vi "Access Privilege_String Encrypt Decrypt.vi"(9 "Encrypted In":u8[][][](array[numeric]), 10 "2D String Data":string[][](array[string])=[["Administrator", "Admin", "Administrator"], ["1", "1", "Administrator"], ["2", "2", "User"]], 11 "Action":enum16{"Encrypt", "Decrypt"}(ring)) -> (1 "Decrypted Out":string[][](array[string]), 2 "Encrypted Out":u8[][][](array[numeric]))   [LabVIEW 2023, in "GUI.lvlib"]
uses:
  GUI.lvlib
  <vilib>/Utility/error.llb/Trim Whitespace One-Sided.vi
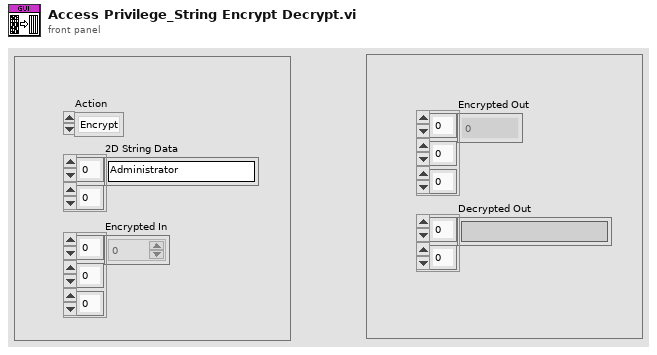
[diagram p1: front panel]
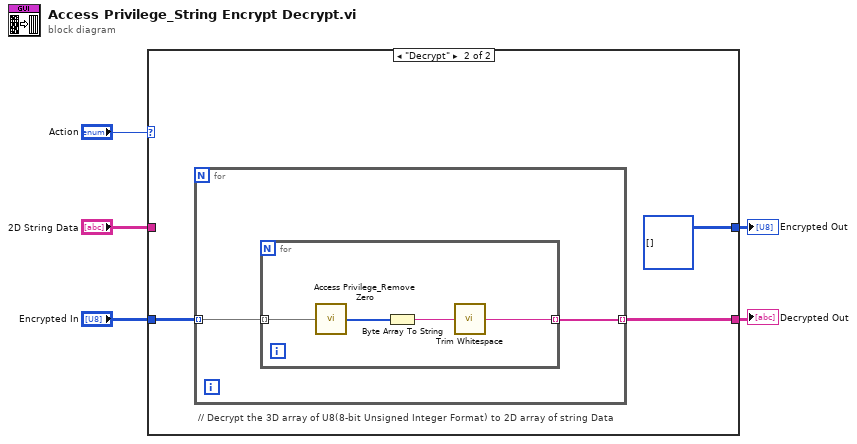
[diagram p0: block diagram]
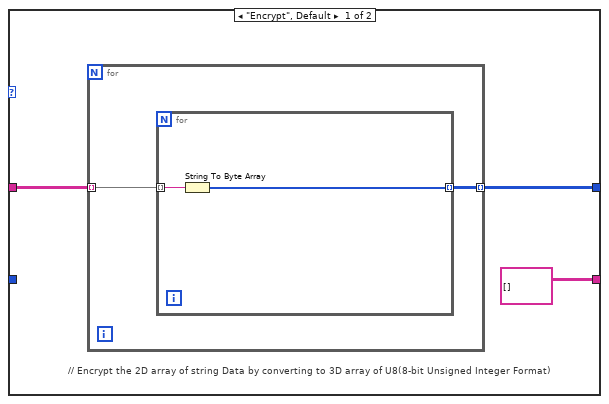
[diagram p2: hidden frame]
diagram:
  n1 = case shown="\"Decrypt\"" "Action" {
    tunnel: "2D String Data" -> [w8 _]
    tunnel: [w7 u8[][][] [] ("unsigned byte array")] -> w3
    tunnel: "Encrypted In" -> [_ w14]
    tunnel: [string[][] [] w13] -> w1
    frame "Encrypt", Default {
      # "// Encrypt the 2D array of string Data by converting to 3D array of U8(8-bit Unsigned Integer Format)"
      n2 = for {
        tunnel: w8 -> [w10] mode=indexing
        tunnel: [w9] -> w7 mode=indexing
        n3 = for {
          tunnel: w10 -> [w12] mode=indexing
          tunnel: [w11] -> w9 mode=indexing
          n4 = String To Byte Array(string=w12) -> (unsigned byte array=w11:u8[])
        }
      }
    }
    frame "Decrypt" {
      # "// Decrypt the 3D array of U8(8-bit Unsigned Integer Format) to 2D array of string Data"
      n5 = for {
        tunnel: w14 -> [w17] mode=indexing
        tunnel: [w16] -> w13 mode=indexing
        n6 = for {
          tunnel: w17 -> [w19] mode=indexing
          tunnel: [w20] -> w16 mode=indexing
          n7 = call "Access Privilege_Remove Zero.vi"("Input Array"=w19) -> ("Output Array"=w18:u8[])  [unwired: 14 in]
          n8 = Byte Array To String(unsigned byte array=w18) -> (string=w21:string)
          n9 = call <vilib>:"Trim Whitespace.vi"("string"=w21) -> ("trimmed string"=w20:string)  [unwired: 1 in]
        }
      }
    }
  }
  "Encrypted Out" <- w3
  "Decrypted Out" <- w1
